vi "status_read.vi"(7 "references":T1, 8 "error in (no error)":errorcluster) -> (0 "error out":errorcluster, 3 "status":T3)   [LabVIEW 2015, in "repub-dvr_nre.lvlib"]
doc: "This VI can be used to read the current status from the module (public). If you want to ensure that you're getting recently updated data rather than the most recent data, you can include a value for timeout. It's default is 0, in the case the default is used, it returns the most recent value (even if it's never been updated). If the timeout is non-zero and there's no new value, it will output a module specific error noting that the status notifier has timed out."
uses:
  repub-dvr_nre.lvlib
  _controls/status.ctl
  lv-recipe-machine/public/_controls/mode.ctl
  lv-recipe-machine/public/_controls/manual_state.ctl
  lv-recipe-machine/public/_controls/automatic_state.ctl
  _controls/references.ctl
  private/_controls/input.ctl
  private/_controls/input_command.ctl
  private/_controls/output.ctl
  private/_controls/data.ctl
  _controls/configuration.ctl
  lv-recipe-machine/private/_controls/recipe_data.ctl
  <userlib>/antonio-alexander/lv-waitgroup/public/_controls/api_waitgroup.ctl
  lv-recipe-machine/public/_controls/transition.ctl
  _controls/change.ctl
  lv-recipe-machine/lv-recipe-machine.lvlib
  <userlib>/antonio-alexander/lv-waitgroup/lv-waitgroup.lvlib
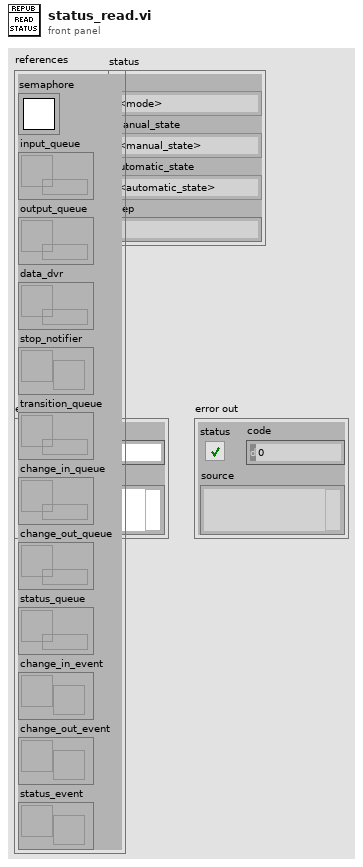
[diagram p1: front panel]
types:
  T1 = typedef "repub-dvr_nre.lvlib/references.ctl" = cluster{"semaphore":T2, "input_queue":refnum<queue>, "output_queue":refnum<queue>, "data_dvr":refnum<data-value>, "stop_notifier":refnum<notifier>, "transition_queue":refnum<queue>, "change_in_queue":refnum<queue>, "change_out_queue":refnum<queue>, "status_queue":refnum<queue>, "change_in_event":refnum<user-event>, "change_out_event":refnum<user-event>, "status_event":refnum<user-event>}
  T2 = typedef "Semaphore RefNum" = refnum<k1>
  T3 = typedef "repub-dvr_nre.lvlib/status.ctl" = cluster{"mode":T4, "manual_state":T5, "automatic_state":T6, "step":string}
  T4 = typedef "lv-recipe-machine.lvlib/mode.ctl" = enum16{"<mode>", "manual", "automatic", "<null>"}
  T5 = typedef "lv-recipe-machine.lvlib/manual_state.ctl" = enum16{"<manual_state>", "failed", "action", "running", "idle", "<null>"}
  T6 = typedef "lv-recipe-machine.lvlib/automatic_state.ctl" = enum16{"<automatic_state>", "failed", "idle", "running", "paused", "transition", "stopped", "<null>"}
  T7 = typedef "repub-dvr_nre.lvlib/data.ctl" = cluster{"configuration":T8, "working":cluster{"recipe_data":T9, "api_waitgroup":T10}}
  T8 = typedef "repub-dvr_nre.lvlib/configuration.ctl" = cluster{dbl}
  T9 = typedef "lv-recipe-machine.lvlib/recipe_data.ctl" = cluster{"mode":T4, "manual_state":T5, "automatic_state":T6, "step":string, "automatic_recipe":variant, "manual_actions":variant}
  T10 = typedef "lv-waitgroup.lvlib/api_waitgroup.ctl" = cluster{"waitgroups":refnum<data-value>, "waitgroup":string}
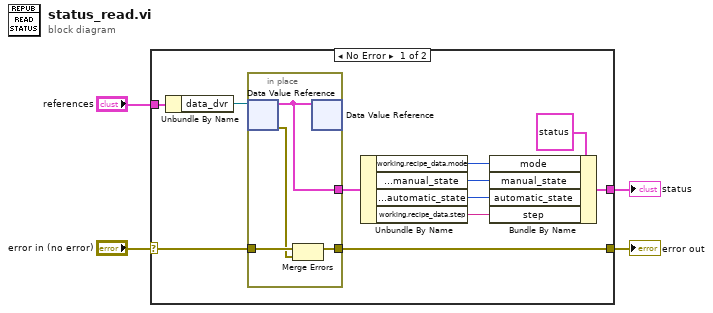
[diagram p0: block diagram]
diagram:
  n1 = case shown="No Error" "error in (no error)" {
    selector: "error in (no error)" -> [w13 w20]
    tunnel: [w12 w20] -> w3
    tunnel: "references" -> [w15 _]
    tunnel: [w10 _] -> w1
    frame No Error {
      n2 = Unbundle By Name(w15) -> ("data_dvr"=w14:refnum<data-value>)
      n3 = in-place {
        in-place-border: w13 -> [w19]
        in-place-border: [w17] -> w12
        in-place-border: [w16] -> w9
        n4 = in-place-dvr #1(w14) -> (w16:T7, w18:errorcluster)
        n5 = Merge Errors(w19, w18) -> (w17:errorcluster)
        n6 = in-place-dvr #1(w16) -> ()  [unwired: 2 out]
      }
      n7 = Unbundle By Name(w9) -> ("working.recipe_data.mode"=w5:T4, "working.recipe_data.manual_state"=w6:T5, "working.recipe_data.automatic_state"=w7:T6, "working.recipe_data.step"=w8:string)
      n8 = Bundle By Name(cluster=T3 {"mode"=enum."<mode>", "manual_state"=enum."<manual_state>", "automatic_state"=enum."<automatic_state>", "step"=""} ("status"), "mode"=w5, "manual_state"=w6, "automatic_state"=w7, "step"=w8) -> (w10:T3)
    }
    frame Error {
    }
  }
  "error out" <- w3
  "status" <- w1
